vi "LinearSystemLoop_New_LinearSystem.vi"(6 "dT_Seconds":dbl, 8 "Max_Voltage":dbl, 9 "Observer":T3, 10 "Controller":T4, 11 "Plant":T1) -> (0 "Error":bool, 3 "Linear System Loop":T5)   [LabVIEW 2019, in "Trajectory_Library.lvlib"]
doc: "Creates a new LINEAR SYSTEM data cluster with the specified values. \n\n\nInputs: \n - XXX -- XXX.\n\nOutputs:\n - XXX -- XXX."
uses:
  Trajectory_Library.lvlib
  LINEAR_SYSTEM.ctl
  <vilib>/Analysis/Matrix/Datatypes/RealMatrix.ctl
  <vilib>/Analysis/Matrix/NI_Matrix.lvlib
  LINEAR_QUADRATIC_REGULATOR.ctl
  LINEAR_PLANT_INV_FF.ctl
  KALMAN_FILTER.ctl
  LINEAR_SYSTEM_LOOP.ctl
panel:
  # "<States,States>"
  # "<States,Inputs>"
  # "<Outputs,States>"
  # "<Outputs,Inputs>"
  # "Steady State Gain  \n<States,Outputs>"
  # "State Estimate <Statess,1>"
  # "<States,States>"
  # "<States,Inputs>"
  # "<Outputs,States>"
  # "<Outputs,Inputs>"
  # "Ref State <States,1>"
  # "Comp and capped \noutput <Inputs,1>"
  # "Controller gain\n<Inputs,States>"
  # "<States,1>"
  # "<FUTURE --- CLAMP TYPE -- For now\nuse Normalize>"
  # "Steady State Gain  \n<States,Outputs>"
  # "State Estimate <Statess,1>"
  # "<States,States>"
  # "<States,Inputs>"
  # "<Outputs,States>"
  # "<Outputs,Inputs>"
  # "<States,1>"
  # "<Inputs,1>"
  # "<States,Inputs>"
  # "<States,States>"
  # "Ref State <States,1>"
  # "Comp and capped \noutput <Inputs,1>"
  # "Controller gain\n<Inputs,States>"
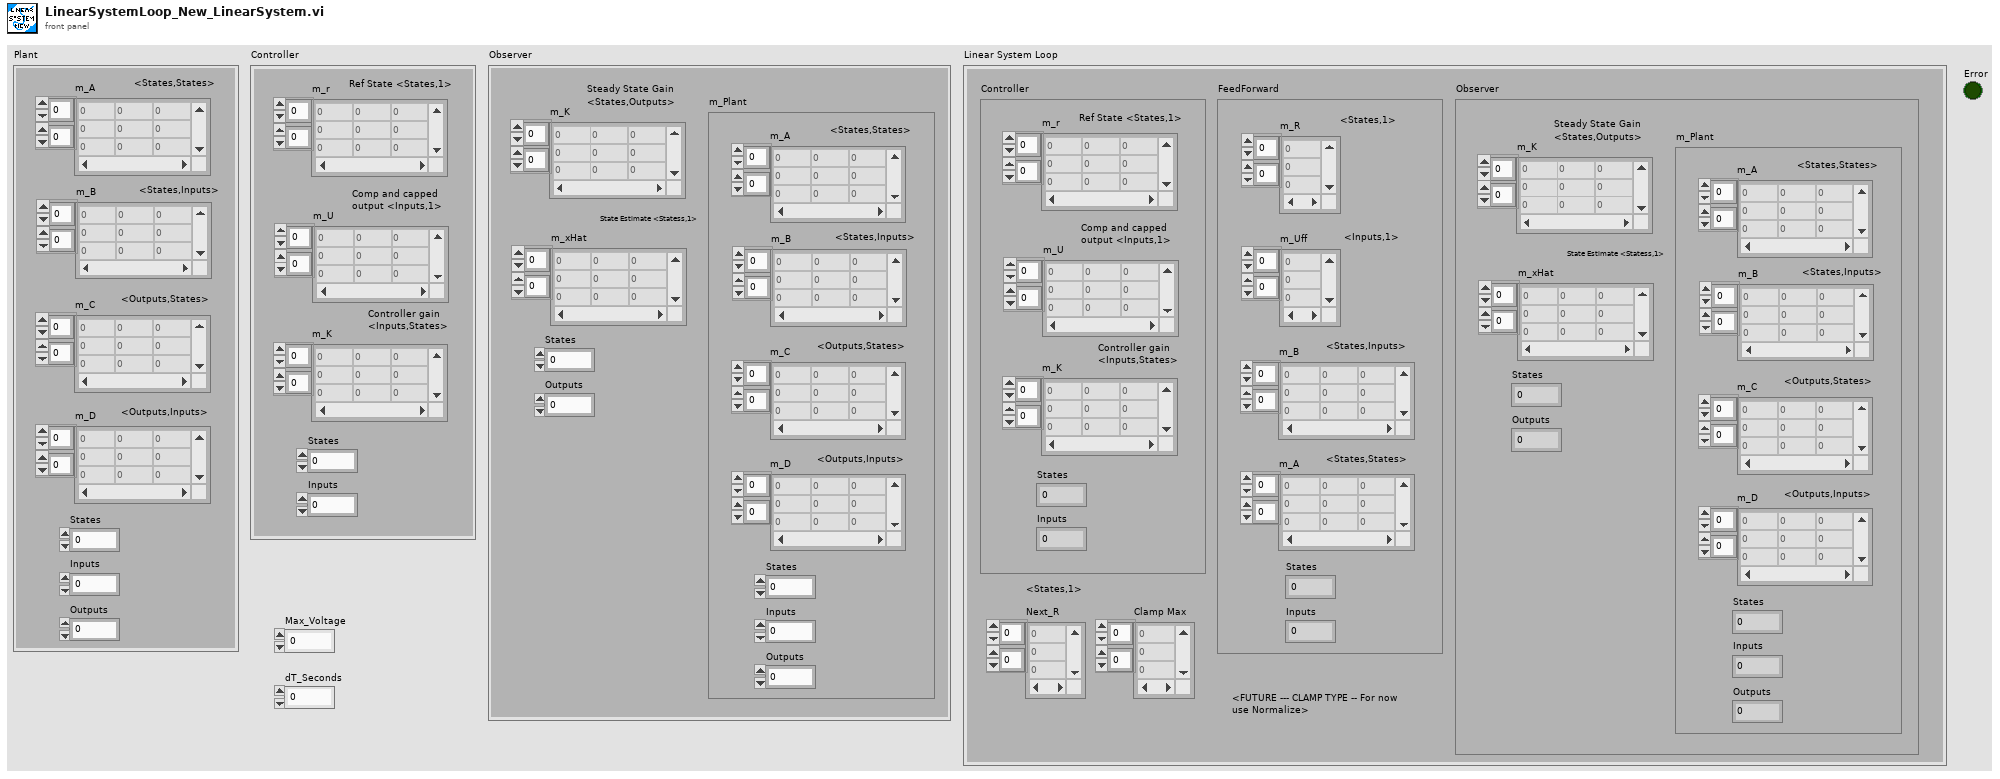
[diagram p1: front panel]
types:
  T1 = typedef "Trajectory_Library.lvlib/LINEAR_SYSTEM.ctl" = cluster{"m_A":T2, "m_B":T2, "m_C":T2, "m_D":T2, "States":i32, "Inputs":i32, "Outputs":i32}
  T2 = typedef "NI_Matrix.lvlib/RealMatrix.ctl" = dbl[][]
  T3 = typedef "Trajectory_Library.lvlib/KALMAN_FILTER.ctl" = cluster{"m_K":T2, "m_xHat":T2, "States":i32, "Outputs":i32, "m_Plant":T1}
  T4 = typedef "Trajectory_Library.lvlib/LINEAR_QUADRATIC_REGULATOR.ctl" = cluster{"m_r":T2, "m_U":T2, "m_K":T2, "States":i32, "Inputs":i32}
  T5 = typedef "Trajectory_Library.lvlib/LINEAR_SYSTEM_LOOP.ctl" = cluster{"Controller":T4, "FeedForward":T6, "Observer":T3, "Next_R":T2, "Clamp Max":T2}
  T6 = typedef "Trajectory_Library.lvlib/LINEAR_PLANT_INV_FF.ctl" = cluster{"m_R":T2, "m_Uff":T2, "m_B":T2, "m_A":T2, "States":i32, "Inputs":i32}
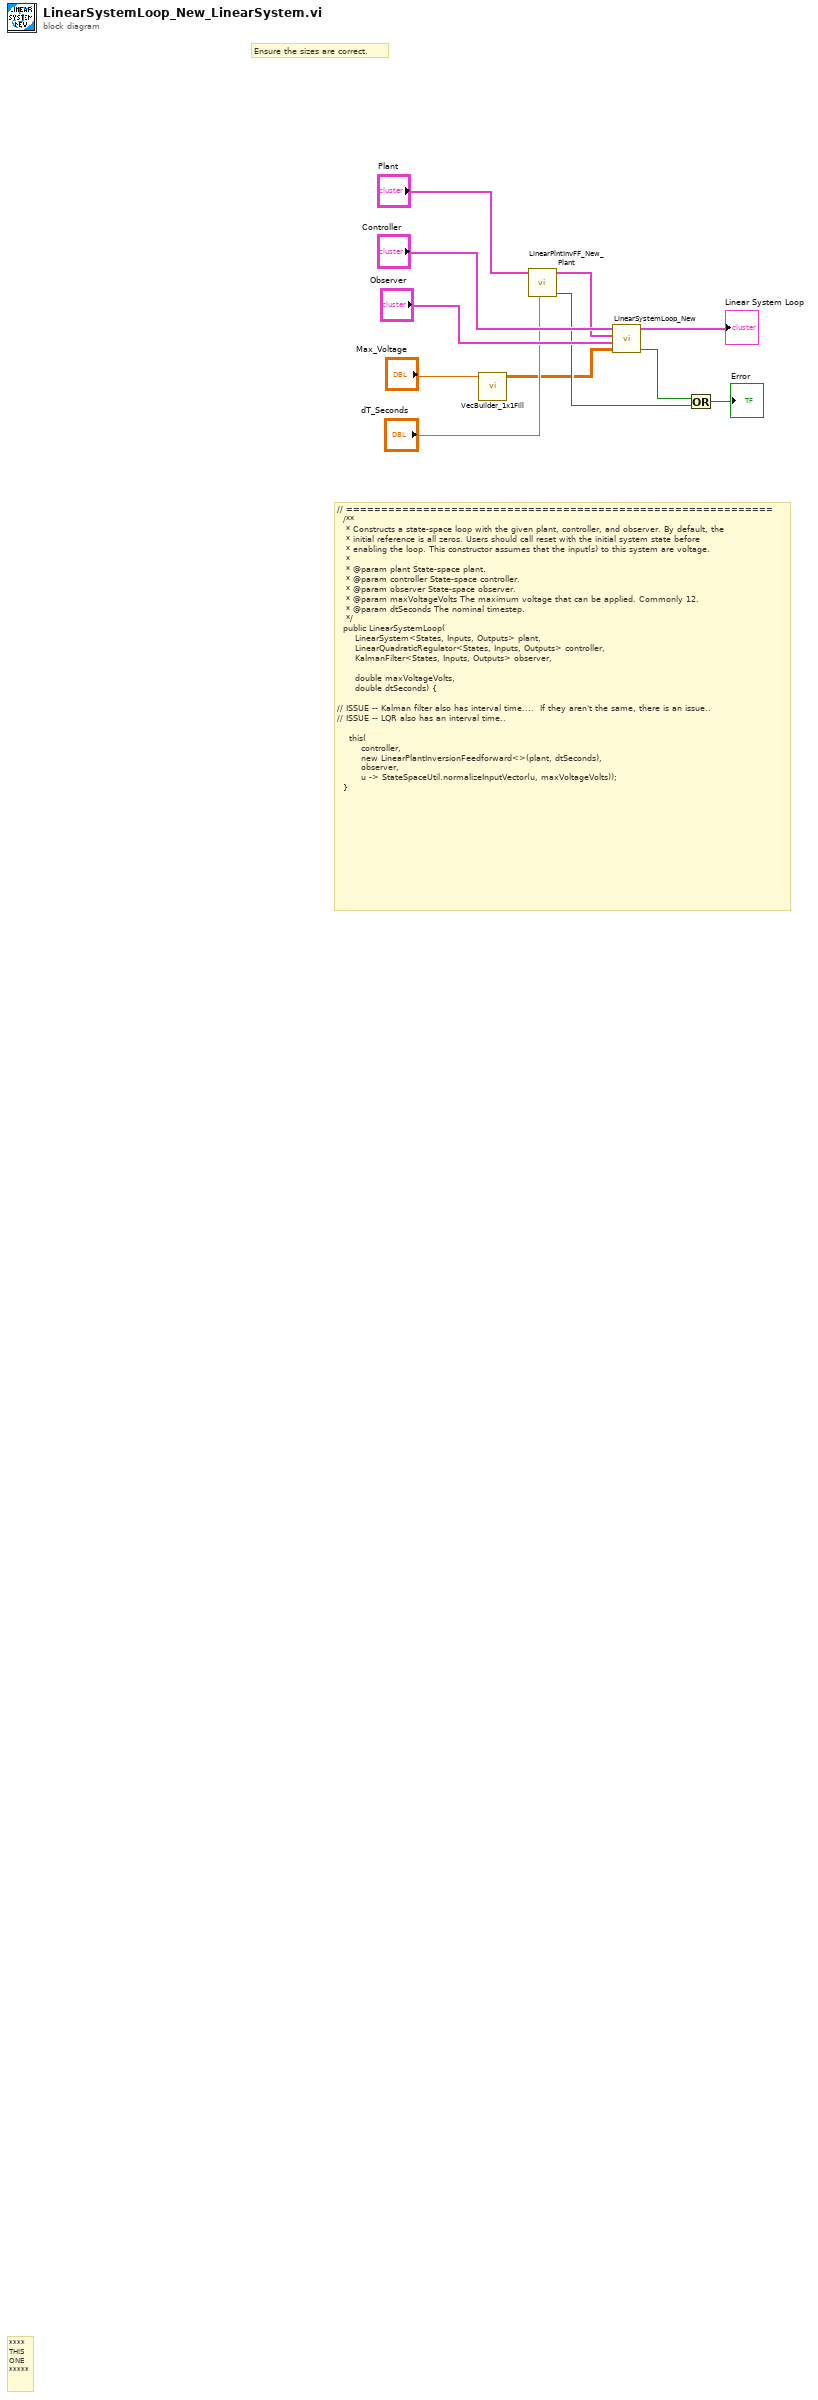
[diagram p0: block diagram]
diagram:
  # "// =============================================================\n  /**\n   * Constructs a state-space loop with the given plant, controller, and observer. By default, the\n   * initial reference is all zeros. Users should call reset with the initial system state before\n   * enabling the loop. This constructor assumes that the input(s) to this system are voltage.\n   *\n   * @param plant State-space plant.\n   * @param controller State-space controller.\n   * @param observer State-space observer.\n   * @param maxVoltageVolts The maximum voltage that can be applied. Commonly 12.\n   * @param dtSeconds The nominal timestep.\n   */\n  public LinearSystemLoop(\n      LinearSystem<States, Inputs, Outputs> plant,\n      LinearQuadraticRegulator<States, Inputs, Outputs> controller,\n      KalmanFilter<States, Inputs, Outputs> observer,\n\n      double maxVoltageVolts,\n      double dtSeconds) {\n\n//\tISSUE -- Kalman filter also has interval time....  If they aren't the same, there is an issue..\n//\tISSUE -- LQR also has an interval time.. \n\n    this(\n        controller,\n        new LinearPlantInversionFeedforward<>(plant, dtSeconds),\n        observer,\n        u -> StateSpaceUtil.normalizeInputVector(u, maxVoltageVolts));\n  }"
  # "Ensure the sizes are correct."
  # "****\nTHIS\nONE\n*****"
  n1 = call "VecBuilder_1x1Fill.vi"("R0_C0"="Max_Voltage") -> ("output matrix"=w2:T2)  [unwired: 10 in]
  n2 = call "LinearPlntInvFF_New_Plant.vi"("dT_Seconds"="dT_Seconds", "Plant"="Plant") -> ("Error"=w4:bool, "Linear Plnt Inversion FF"=w5:T6)  [unwired: 8 in]
  n3 = call "LinearSystemLoop_New.vi"("Max Input"=w2, "Observer"="Observer", "FeedForward"=w5, "Controller"="Controller") -> ("Error"=w6:bool, "Linear System Loop"=→"Linear System Loop":T5)  [unwired: 6 in]
  n4 = Or(x=w6, y=w4) -> (x .or. y?=→"Error":bool)
